vi "Publish Data.vi"(8 "error passthrough":errorcluster, 11 "Module Data In":refnum<class "Rename.lvclass">) -> (0 "error passthrough":errorcluster, 3 "Module Data Out":refnum<class "Rename.lvclass">)   [LabVIEW 2015, in "Generic Module Library.lvlib" / "Template G_Module.lvlib"]
uses:
  Template G_Module.lvlib
  Module Data Access/Data Access Support/Data Actions.ctl
  Module Class/Rename.lvclass
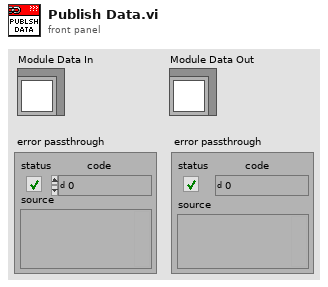
[diagram p1: front panel]
types:
  T1 = typedef "Generic Module Library.lvlib/Template G_Module.lvlib/Data Actions.ctl" = enum16{"Set", "Get"}
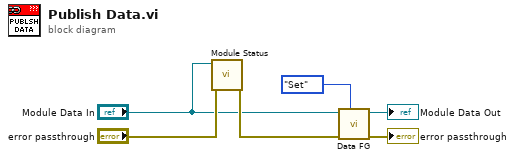
[diagram p0: block diagram]
diagram:
  n1 = call "Module Status.vi"("error in"="error passthrough", "Module Data In"="Module Data In") -> ("error out"=w2:errorcluster)  [unwired: 9 in]
  n2 = call "Data FG.vi"("Data Action"=Data_Actions."Set", "error in (no error)"=w2, "Data In"="Module Data In") -> ("error out"=→"error passthrough":errorcluster, "Data Out"=→"Module Data Out":refnum<class "Rename.lvclass">)  [unwired: 7 in]
